vi "1WIRE_Read_Byte_multi.vi"(8 "error in":errorcluster, 11 "FPGA I/O":refnum<k21>="DS_WIRE") -> (0 "error out":errorcluster, 2 "Array":bool[](array[boolean]))   [LabVIEW 2012]
doc: "This VI is created by Vincent Claes for FPDA-1 more information on http://pwo.fpga.be\n\nvincent.claes@xios.be\nclaesvincent@gmail.com\n\nhttp://www.linkedin.com/in/vincentclaes"
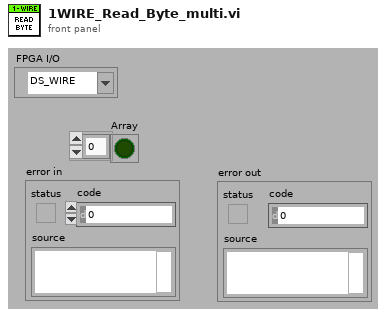
[diagram p1: front panel]
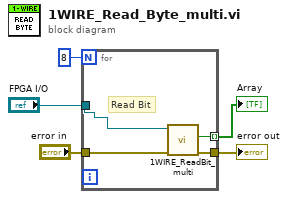
[diagram p0: block diagram]
diagram:
  n1 = for {
    N: 8 -> [_]
    tunnel: [w9] -> w5 mode=indexing
    tunnel: "error in" -> [w8]
    tunnel: [w7] -> w2
    tunnel: "FPGA I/O" -> [w6]
    # "Read Bit"
    n2 = call "1WIRE_ReadBit_multi.vi"("error in"=w8, "FPGA I/O"=w6) -> ("error out"=w7:errorcluster, "Bit Read"=w9:bool)  [unwired: 8 in]
  }
  "Array" <- w5
  "error out" <- w2
